vi "Show UI.vi"(8 "error in (no error)":errorcluster, 11 "Actor wUI in":refnum<class "Actor wUI.lvclass">) -> (0 "error out":errorcluster, 3 "Actor wUI out":refnum<class "Actor wUI.lvclass">)   [LabVIEW 2017, in "Framework.lvlib" / "Actor wUI.lvclass"]
uses:
  Actor wUI.lvclass
  Actor wUI.lvclass/Actor wUI.ctl
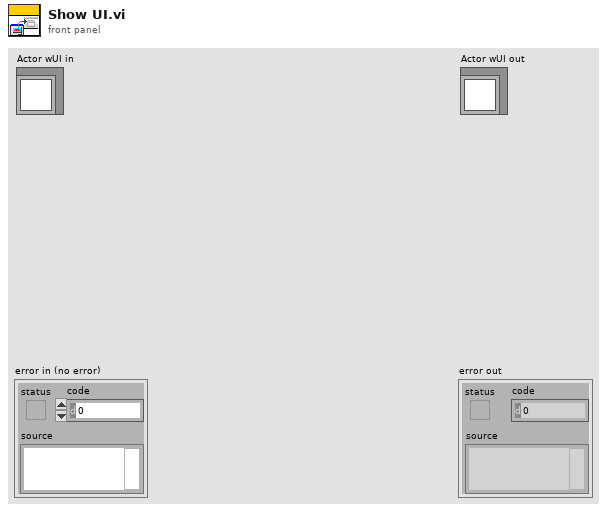
[diagram p1: front panel]
types:
  T1 = enum32{"Invalid", "Standard", "Closed", "Hidden", "Minimized", "Maximized"}
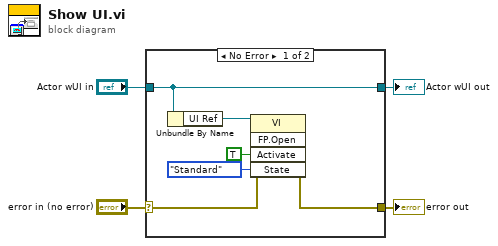
[diagram p0: block diagram]
diagram:
  n1 = case shown="No Error" "error in (no error)" {
    selector: "error in (no error)" -> [w6 w12]
    tunnel: [w5 w12] -> w3
    tunnel: [w10 w11] -> w1
    tunnel: "Actor wUI in" -> [w10 w11]
    frame No Error {
      n2 = Unbundle By Name(w10) -> ("UI Ref"=w9:refnum<vi>)
      n3 = invoke class="VI" method="FP.Open"(reference=w9, error in=w6, "Activate"=TRUE ("Activate?"), "State"=T1."Standard") -> (error out=w5:errorcluster)  [unwired: 1 in, 4 out]
    }
    frame Error {
    }
  }
  "error out" <- w3
  "Actor wUI out" <- w1
